vi "Dark Correct.vi"(7 "Dark Array Path":path=path "C:/Users/dhstuart/Dropbox/CLTC/avantesSpectrometer/Cal Files/Dark Model Parameters.csv", 8 "error in (no error)":errorcluster, 9 "Counts":dbl[](array[numeric]), 11 "AVS Settings In":T1) -> (0 "error out":errorcluster, 1 "Counts normalize and dark corrected":dbl[](array[numeric]), 3 "AVS Settings Out":T1)   [LabVIEW 2013]
uses:
  Libraries/AS-5216-DLL/AVS settings.ctl
  <vilib>/Analysis/1siggen.llb/Ramp Pattern by Delta.vi
  <vilib>/Utility/file.llb/Read From Spreadsheet File (DBL).vi
  <vilib>/express/express arith-compare/Formula/XNode/ExpressFormulaBlockNode.xnode
  <vilib>/Analysis/NI_AALBase.lvlib
  AvaSpec.lvlib
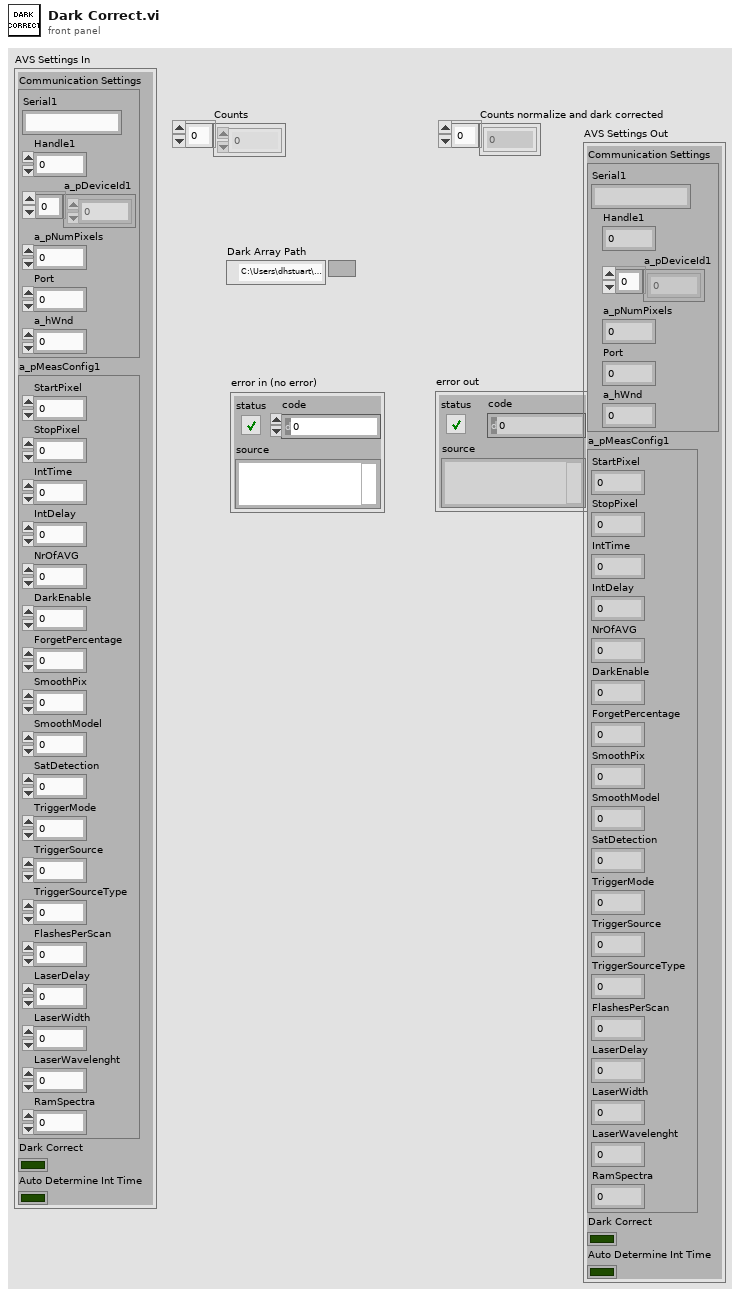
[diagram p1: front panel]
types:
  T1 = typedef "AvaSpec.lvlib/AVS settings.ctl" = cluster{"Communication Settings":cluster{"Serial1":string, "Handle1":i32, "a_pDeviceId1":u8[], "a_pNumPixels":u16, "Port":i32, "a_hWnd":i32}, "a_pMeasConfig1":cluster{"StartPixel":u16, "StopPixel":u16, "IntTime":sgl, "IntDelay":u32, "NrOfAVG":u32, "DarkEnable":u8, "ForgetPercentage":u8, "SmoothPix":u16, "SmoothModel":u8, "SatDetection":u8, "TriggerMode":u8, "TriggerSource":u8, "TriggerSourceType":u8, "FlashesPerScan":u16, "LaserDelay":u32, "LaserWidth":u32, "LaserWavelenght":sgl, "RamSpectra":u16}, "Dark Correct":bool, "Auto Determine Int Time":bool}
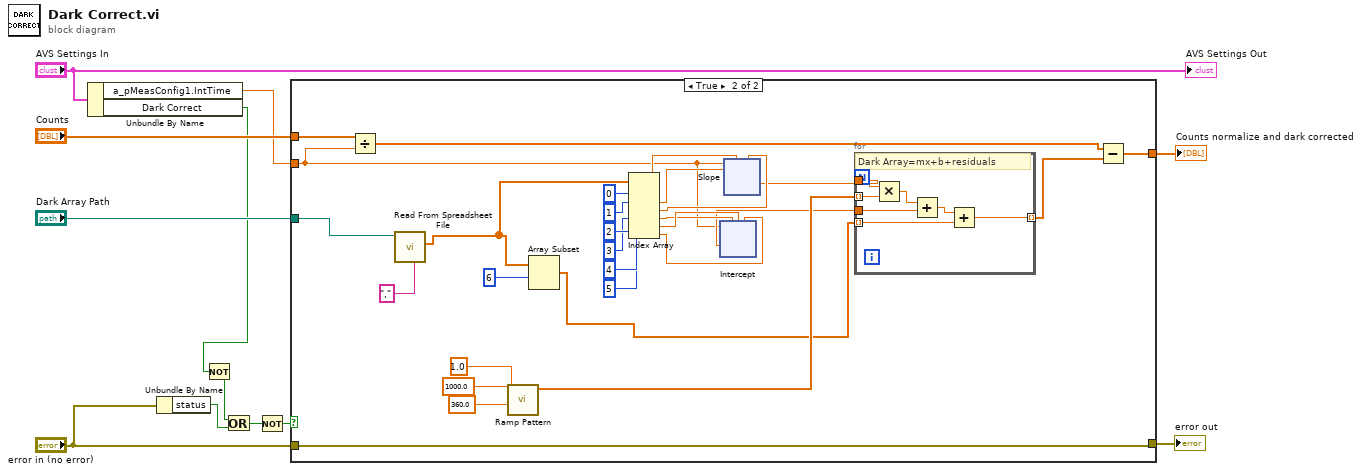
[diagram p0: block diagram]
diagram:
  n1 = Unbundle By Name("AVS Settings In") -> ("a_pMeasConfig1.IntTime"=w7:sgl, "Dark Correct"=w4:bool)
  n2 = Unbundle By Name("error in (no error)") -> ("status"=w5:bool)
  n3 = Not(x=w4) -> (.not. x?=w3:bool)
  n4 = Or(x=w3, y=w5) -> (x .or. y?=w1:bool)
  n5 = Not(x=w1) -> (.not. x?=w2:bool)
  n6 = case shown="True" w2 {
    tunnel: "Dark Array Path" -> [_ w24]
    tunnel: w7 -> [_ w22]
    tunnel: "Counts" -> [w14 w23]
    tunnel: [w14 w19] -> w10
    tunnel: [w13 w15] -> w9
    tunnel: "error in (no error)" -> [w13 w15]
    frame False {
    }
    frame True {
      n7 = Divide(x=w23, y=w22) -> (x/y=w21:dbl[])
      n8 = call-poly <vilib>:"Read From Spreadsheet File.vi"("delimiter (\\t)"="," ("delimiter (\\t)"), "file path (dialog if empty)"=w24) -> ("first row"=w18:dbl[])  [unwired: 5 in, 4 out]
      n9 = call-poly <vilib>:"Ramp Pattern.vi"("start"=360.0, "end"=1000.0, "delta"=1.0) -> ("Ramp Pattern"=w27:dbl[])  [unwired: 6 in, 2 out]
      n10 = Array Subset(array=w18, index=6) -> (w17:dbl[])  [unwired: 1 in]
      n11 = Index Array(array=w18, index #1=0 ("index"), index #2=1 ("index"), index #3=2 ("index"), index #4=3 ("index"), index #5=4 ("index"), index #6=5 ("index")) -> (element #1=w36:dbl, element #2=w35:dbl, element #3=w34:dbl, element #4=w31:dbl, element #5=w32:dbl, element #6=w33:dbl)
      n12 = xnode "Intercept"("intTime"=w22, "a"=w31, "b"=w32, "c"=w33) -> ("Result"=w25:dbl)  [unwired: 1 in, 1 out]
      n13 = xnode "Slope"("intTime"=w22, "a"=w36, "b"=w35, "c"=w34) -> ("Result"=w26:dbl)  [unwired: 1 in, 1 out]
      n14 = for {
        tunnel: w17 -> [w45] mode=indexing
        tunnel: w27 -> [w49] mode=indexing
        tunnel: w26 -> [w50]
        tunnel: w25 -> [w47]
        tunnel: [w44] -> w20 mode=indexing
        # "Dark Array=mx+b+residuals"
        n15 = Multiply(x=w50, y=w49) -> (x*y=w48:dbl)
        n16 = Add(x=w48, y=w47) -> (x+y=w46:dbl)
        n17 = Add(x=w46, y=w45) -> (x+y=w44:dbl)
      }
      n18 = Subtract(x=w21, y=w20) -> (x-y=w19:dbl[])
    }
  }
  "error out" <- w9
  "Counts normalize and dark corrected" <- w10
  "AVS Settings Out" <- "AVS Settings In"
